vi "GT Arc XYC.vi"(0 "cardNum":i16, 1 "crd":i16, 3 "x":i32, 4 "y":i32, 5 "error in (no error)":errorcluster caption="错误输入（无错误）", 6 "xCenter":dbl, 7 "yCenter":dbl, 8 "fifo":i16, 10 "circleDir":i16(ring) items=["0：顺时针圆弧。", "1：逆时针圆弧"], 11 "synVel":dbl, 12 "synAcc":dbl, 13 "velEnd":dbl) -> (14 "function return":i16, 19 "error out":errorcluster caption="错误输出")   [LabVIEW 2020, in "gts.lvlib"]
doc: "GT_API GT_ArcXYC(short cardNum,short crd,long x,long y,double xCenter,double yCenter,short circleDir,double synVel,double synAcc,double velEnd=0,short fifo=0);\n\ncrd 坐标系号。正整数，取值范围：[1, 2]。 x 圆弧插补 x 轴的终点坐标值。取值范围：[-1073741823, 1073741823]，单位：pulse。 y 圆弧插补 y 轴的终点坐标值。取值范围：[-1073741823, 1073741823]，单位：pulse。\nxCenter 圆弧插补的圆心 x 方向相对于起点位置的偏移量。\nyCenter 圆弧插补的圆心 y 方向相对于起点位置的偏移量。\ncircleDir\n圆弧的旋转方向。 0：顺时针圆弧。1：逆时针圆弧。\nsynVel 插补段的目标合成速度。取值范围：(0, 32767)，单位：pulse/ms。\nsynAcc 插补段的合成加速度。取值范围：(0, 32767)，单位：pulse/ms2。\nvelEnd\n插补段的终点速度。取值范围：[0, 32767)，单位：pulse/ms。该值只有在没有使用\n前瞻预处理功能时才有意义，否则该值无效。默认值为：0。\nfifo 插补缓存区号。正整数，取值范围：[0, 1]，默认值为：0。\n指令返回值\n若返回值为 1：\n(1) 检查当前坐标系是否映射了相关轴。\n(2) 检查是否向 fifo1 中传递数据，若是，则检查 fifo0 是否使用并运动，若运动，\n则返回错误。\n(3) 检查相应的 fifo 是否已满。"
uses:
  gts.lvlib
  dll/32bit/multi_card/gts.dll
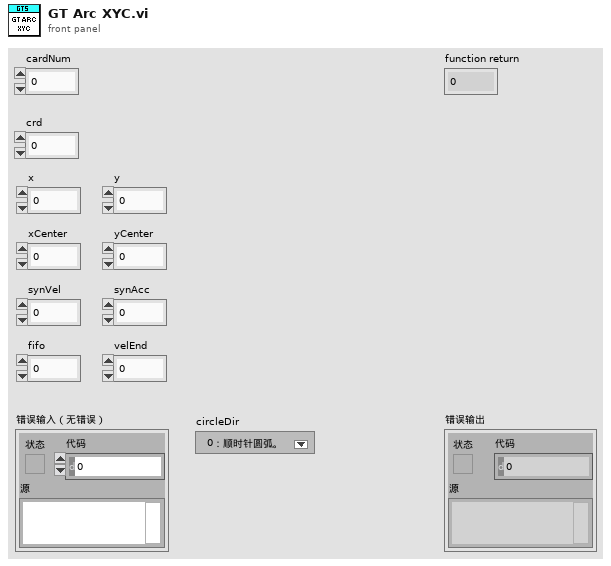
[diagram p1: front panel]
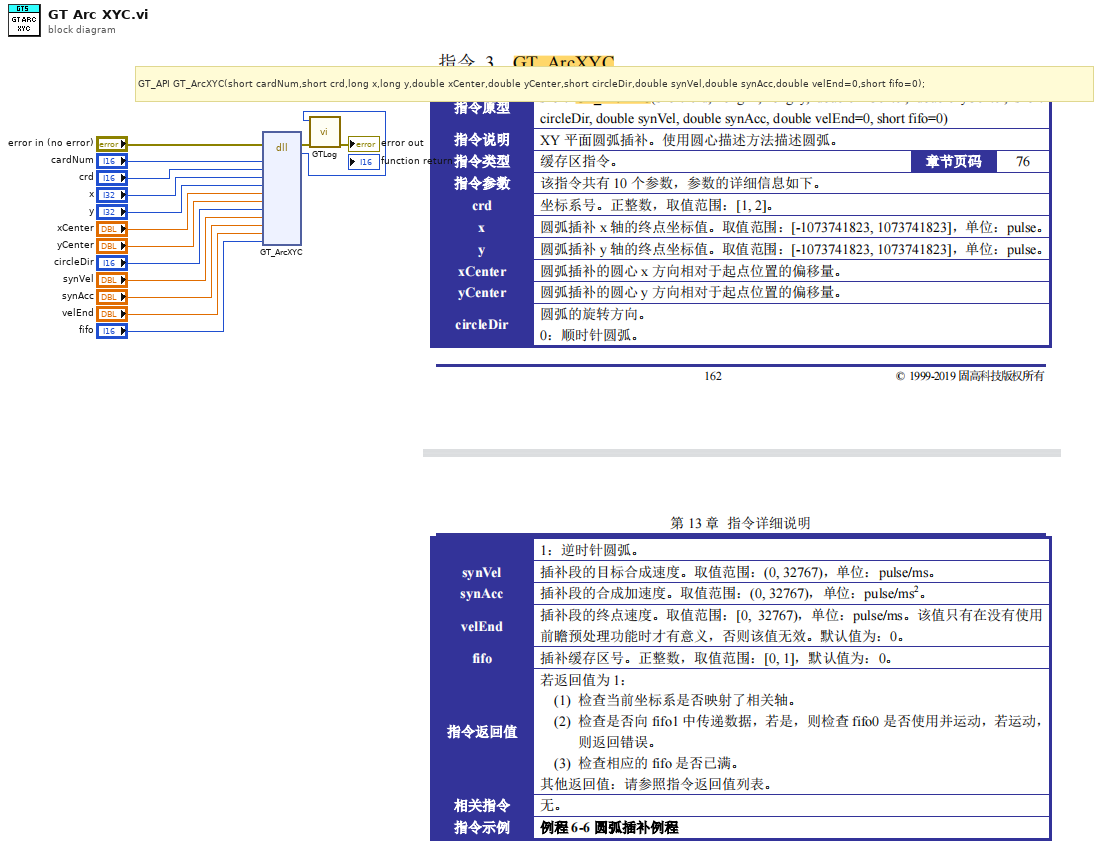
[diagram p0: block diagram]
diagram:
  # "GT_API GT_ArcXYC(short cardNum,short crd,long x,long y,double xCenter,double yCenter,short circleDir,double synVel,double synAcc,double velEnd=0,short fifo=0);"
  n1 = dll-call lib="C:/1228/dll/32bit/multi_card/gts.dll" fn="GT_ArcXYC"(error in="error in (no error)", "cardNum"="cardNum", "crd"="crd", "x"="x", "y"="y", "xCenter"="xCenter", "yCenter"="yCenter", "circleDir"="circleDir", "synVel"="synVel", "synAcc"="synAcc", "velEnd"="velEnd", "fifo"="fifo") -> (error out=w3:errorcluster, w1:i16)  [unwired: 13 in, 1 out]
  n2 = call "GTLog.vi"("error in (no error)"=w3, "Numeric"=w1) -> ("error out"=→"error out":errorcluster)  [unwired: 9 in]
